vi "Update Time.vi"(8 "error in (no error)":errorcluster, 10 "Timestamp":timestamp, 11 "Example View In":refnum<class "Example GUI View.lvclass">) -> (0 "error out":errorcluster, 3 "Example View Out":refnum<class "Example GUI View.lvclass">)   [LabVIEW 2023, in "Example GUI View.lvlib" / "Example GUI View.lvclass"]
uses:
  Example GUI View.lvclass
  Example GUI View.lvclass/Example GUI View.ctl
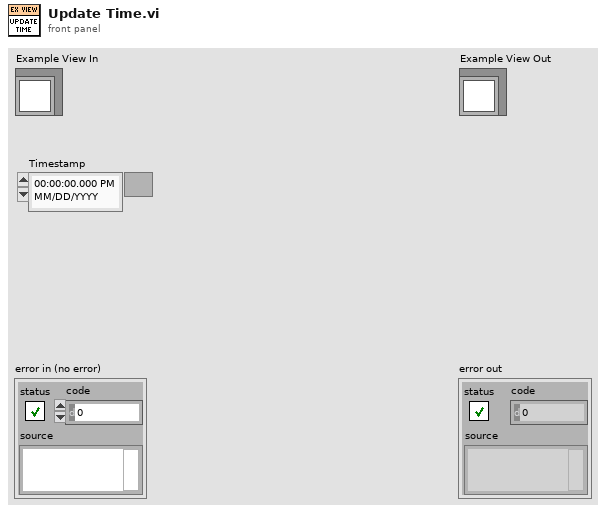
[diagram p1: front panel]
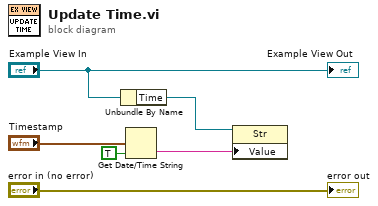
[diagram p0: block diagram]
diagram:
  n1 = Unbundle By Name("Example View In") -> ("Time"=w4:refnum<vi>)
  n2 = Get Date/Time String(seconds (now)="Timestamp", want seconds? (F)=TRUE) -> (time string=w3:string)  [unwired: 1 in, 1 out]
  n3 = property class="Str"(reference=w4, "Value"=w3) -> ()  [unwired: 1 in, 2 out]
  "error out" <- "error in (no error)"
  "Example View Out" <- "Example View In"
